vi "AWS-S3-DestroyClient.vi"(0 "AWS-S3-API":refnum<class "AWS-S3-API.lvclass">, 11 "error in":errorcluster) -> (15 "error out":errorcluster)   [LabVIEW 2012, in "AWS-S3-API.lvclass"]
uses:
  AWS-S3-API.lvclass
  C:/Users/Jack/repo/visualize/Dependencies/aws/AWS-SDK/AWSSDK.dll
  AWS-SDK/AWSSDK.dll
  AWS-S3-API.lvclass/AWS-S3-API.ctl
panel:
  # "Inputs"
  # "Outputs"
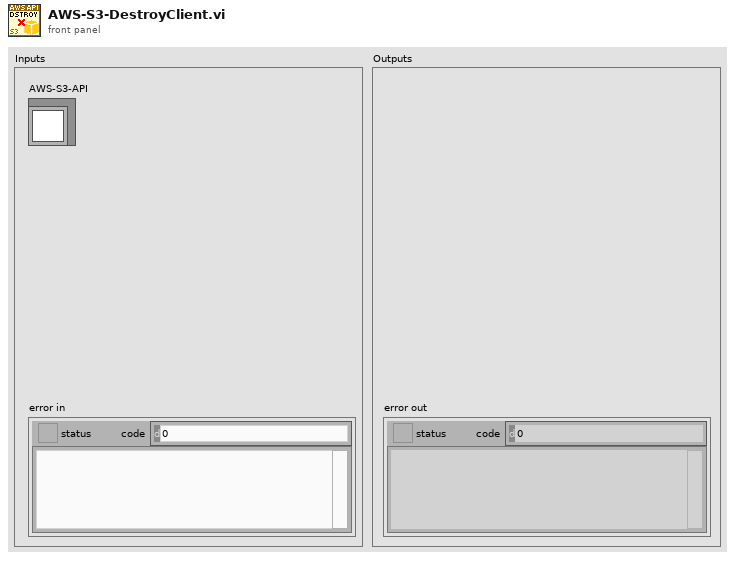
[diagram p1: front panel]
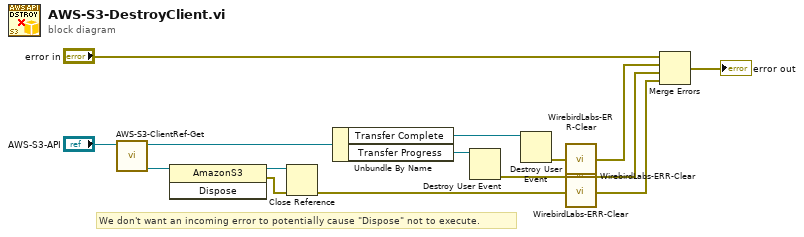
[diagram p0: block diagram]
diagram:
  # "We don't want an incoming error to potentially cause \"Dispose\" not to execute."
  n1 = call "AWS-S3-ClientRef-Get.vi"("AWS-S3-API"="AWS-S3-API") -> ("S3 Client ref"=w9:refnum<k24>, "AWS-S3-API out"=w7:refnum<class "AWS-S3-API.lvclass">)  [unwired: 9 in]
  n2 = invoke class="AmazonS3" method="Dispose"(reference=w9) -> (reference out=w12:refnum<k24>, error out=w11:errorcluster)  [unwired: 2 in, 1 out]
  n3 = Close Reference(reference=w12, error in (no error)=w11) -> (error out=w2:errorcluster)
  n4 = Unbundle By Name(w7) -> ("Transfer Complete"=w10:refnum<user-event>, "Transfer Progress"=w13:refnum<user-event>)
  n5 = Destroy User Event(user event=w13) -> (error out=w5:errorcluster)  [unwired: 1 in]
  n6 = Destroy User Event(user event=w10) -> (error out=w6:errorcluster)  [unwired: 1 in]
  n7 = call "WirebirdLabs-ERR-Clear.vi"("error to snuff"=w6) -> ("no error"=w3:errorcluster)
  n8 = call "WirebirdLabs-ERR-Clear.vi"("error to snuff"=w5) -> ("no error"=w4:errorcluster)
  n9 = call "WirebirdLabs-ERR-Clear.vi"("error to snuff"=w2) -> ("no error"=w1:errorcluster)
  n10 = Merge Errors("error in", w3, w4, w1) -> (→"error out":errorcluster)
